vi "getEventSelection.vi"(8 "error in (no error)":errorcluster, 10 "selectedIndex":i32, 11 "ScriptEventList in":refnum<class "ScriptEventList.lvclass">) -> (0 "error out":errorcluster, 2 "indexArray":i32[](array[numeric]), 3 "ScriptEventList out":refnum<class "ScriptEventList.lvclass">)   [LabVIEW 2011, in "Tools.lvlib" / "Scripting.lvlib" / "ScriptEventList.lvclass"]
uses:
  ScriptEventList.lvclass
  ScriptEventList.lvclass/ScriptEventList.ctl
  ScriptEvent.lvclass
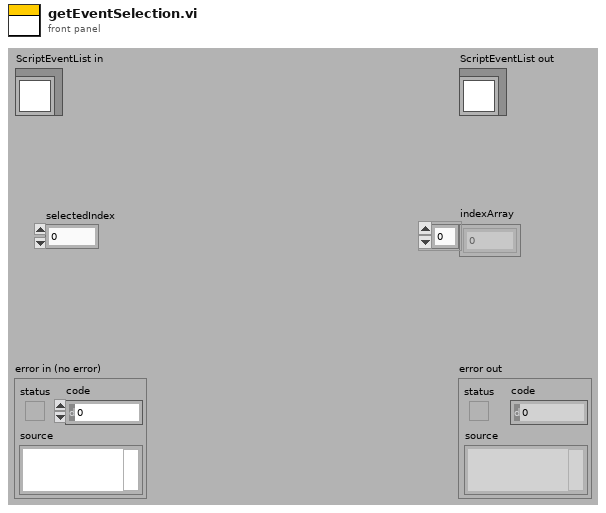
[diagram p1: front panel]
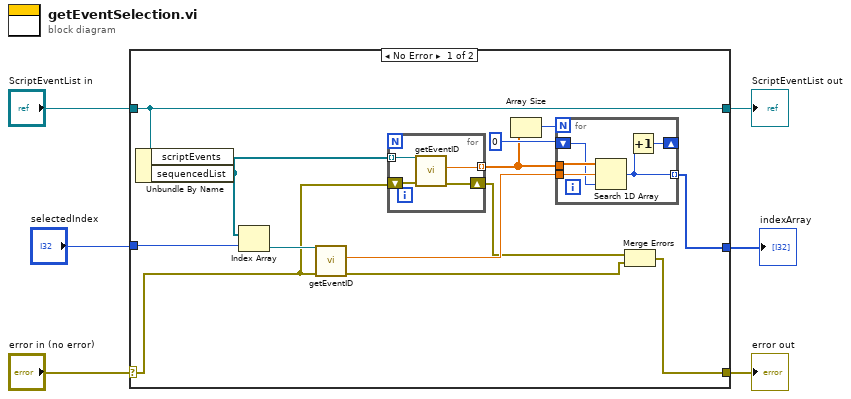
[diagram p0: block diagram]
diagram:
  n1 = case shown="No Error" "error in (no error)" {
    selector: "error in (no error)" -> [w16 w30]
    tunnel: [w12 w30] -> w1
    tunnel: [w19 w29] -> w2
    tunnel: "ScriptEventList in" -> [w19 w29]
    tunnel: "selectedIndex" -> [w18 _]
    tunnel: [w8 _] -> w4
    frame No Error {
      n2 = Unbundle By Name(w19) -> ("sequencedList"=w7:refnum<class "ScriptEvent.lvclass">[])  [unwired: 1 out]
      n3 = Index Array(array=w7, index=w18) -> (element=w17:refnum<class "ScriptEvent.lvclass">)
      n4 = call "getEventID.vi"("error in (no error)"=w16, "ScriptEvent in"=w17) -> ("error out"=w13:errorcluster, "eventId"=w15:dbl)  [unwired: 7 in, 1 out]
      n5 = for {
        tunnel: w7 -> [w28] mode=indexing
        tunnel: [w26] -> w9 mode=indexing
        shift-right: [w25] -> w14
        shift-left: w16 -> [w27]
        n6 = call "getEventID.vi"("error in (no error)"=w27, "ScriptEvent in"=w28) -> ("error out"=w25:errorcluster, "eventId"=w26:dbl)  [unwired: 7 in, 1 out]
      }
      n7 = Array Size(array=w9) -> (size(s)=w10:i32)
      n8 = for {
        N: w10 -> [_]
        tunnel: w9 -> [w23]
        tunnel: w15 -> [w24]
        tunnel: [w22] -> w8 mode=indexing
        shift-right: [w20] -> _
        shift-left: 0 -> [w21]
        n9 = Search 1D Array(1D array=w23, element=w24, start index (0)=w21) -> (index of element=w22:i32)
        n10 = Increment(x=w22) -> (x+1=w20:i32)
      }
      n11 = Merge Errors(w14, w13) -> (w12:errorcluster)
    }
    frame Error {
    }
  }
  "error out" <- w1
  "ScriptEventList out" <- w2
  "indexArray" <- w4
